vi "LED ON AND OFF.vi"() -> ()   [LabVIEW 2012]
panel:
  out "Boolean":bool
  in  "Numeric":dbl
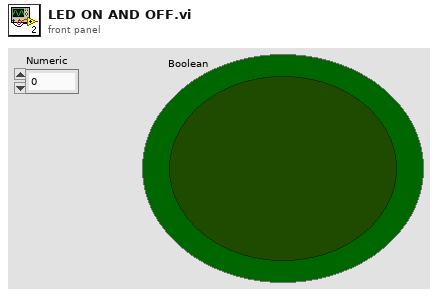
[diagram p1: front panel]
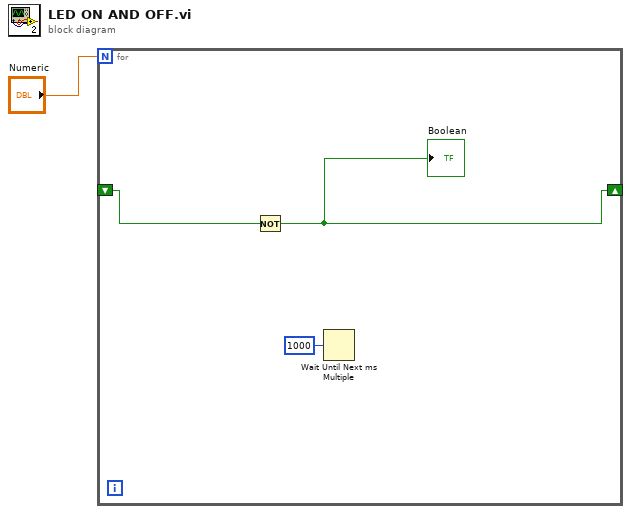
[diagram p0: block diagram]
diagram:
  n1 = for {
    N: "Numeric" -> [_]
    shift-right: [w3] -> _
    shift-left: _ -> [w4]
    n2 = Not(x=w4) -> (.not. x?=w3:bool)
    "Boolean" <- w3
    n3 = Wait Until Next ms Multiple(millisecond multiple=u32 1000) -> ()  [unwired: 1 out]
  }
